vi "Create Temporary Root Folder.vi"(8 "Error In":errorcluster, 11 "Folder Names":string[](array[string])) -> (0 "Error Out":errorcluster, 3 "Temp Log Folder":path)   [LabVIEW 2015, in "Logger.lvlib"]
uses:
  Logger.lvlib
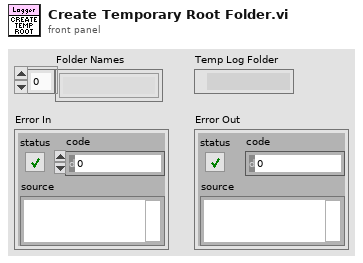
[diagram p1: front panel]
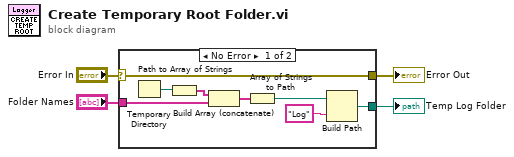
[diagram p0: block diagram]
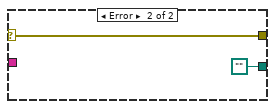
[diagram p2: hidden frame]
diagram:
  n1 = case shown="No Error" "Error In" {
    selector: "Error In" -> [w5 w14]
    tunnel: "Folder Names" -> [w10 _]
    tunnel: [w6 path ""] -> w3
    tunnel: [w5 w14] -> w1
    frame No Error {
      n2 = Temporary Directory() -> (w12:path)
      n3 = Path to Array of Strings(0:w12) -> (2:w11:string[])  [unwired: 1 out]
      n4 = Build Array (concatenate)(w11, w10) -> (w9:string[])
      n5 = Array of Strings to Path(0:w9) -> (2:w8:path)  [unwired: 1 in]
      n6 = Build Path(base path=w8, name or relative path="Log") -> (appended path=w6:path)
    }
    frame Error {
    }
  }
  "Temp Log Folder" <- w3
  "Error Out" <- w1
